vi "题目二.vi"() -> ()   [LabVIEW 2017]
panel:
  out "波形图":dbl[][](graph)
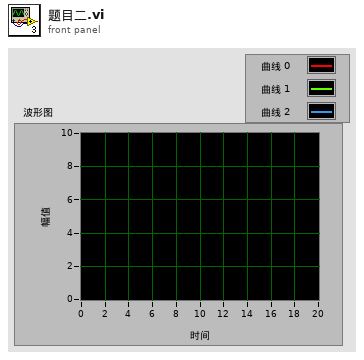
[diagram p1: front panel]
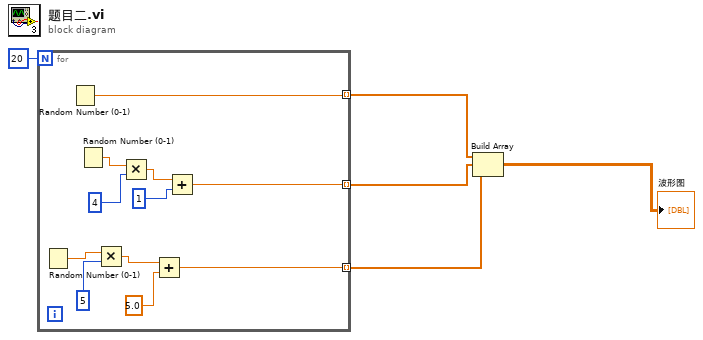
[diagram p0: block diagram]
diagram:
  n1 = for {
    N: 20 -> [_]
    tunnel: [w8] -> w5 mode=indexing
    tunnel: [w7] -> w4 mode=indexing
    tunnel: [w6] -> w3 mode=indexing
    n2 = Random Number (0-1)() -> (number: 0 to 1=w12:dbl)
    n3 = Random Number (0-1)() -> (number: 0 to 1=w8:dbl)
    n4 = Random Number (0-1)() -> (number: 0 to 1=w16:dbl)
    n5 = Multiply(x=w12, y=5) -> (x*y=w10:dbl)
    n6 = Multiply(x=w16, y=4) -> (x*y=w14:dbl)
    n7 = Add(x=w10, y=5.0) -> (x+y=w6:dbl)
    n8 = Add(x=w14, y=1) -> (x+y=w7:dbl)
  }
  n9 = Build Array(w5, w4, w3) -> (→"波形图":dbl[][])
